vi "Change map display.vi"(9 "robot direction":string, 10 "robot location":dbl[](array[numeric]), 11 "Display Map":dbl[][](array[numeric])) -> (3 "New Display Map":dbl[][](array[numeric]))   [LabVIEW 2015]
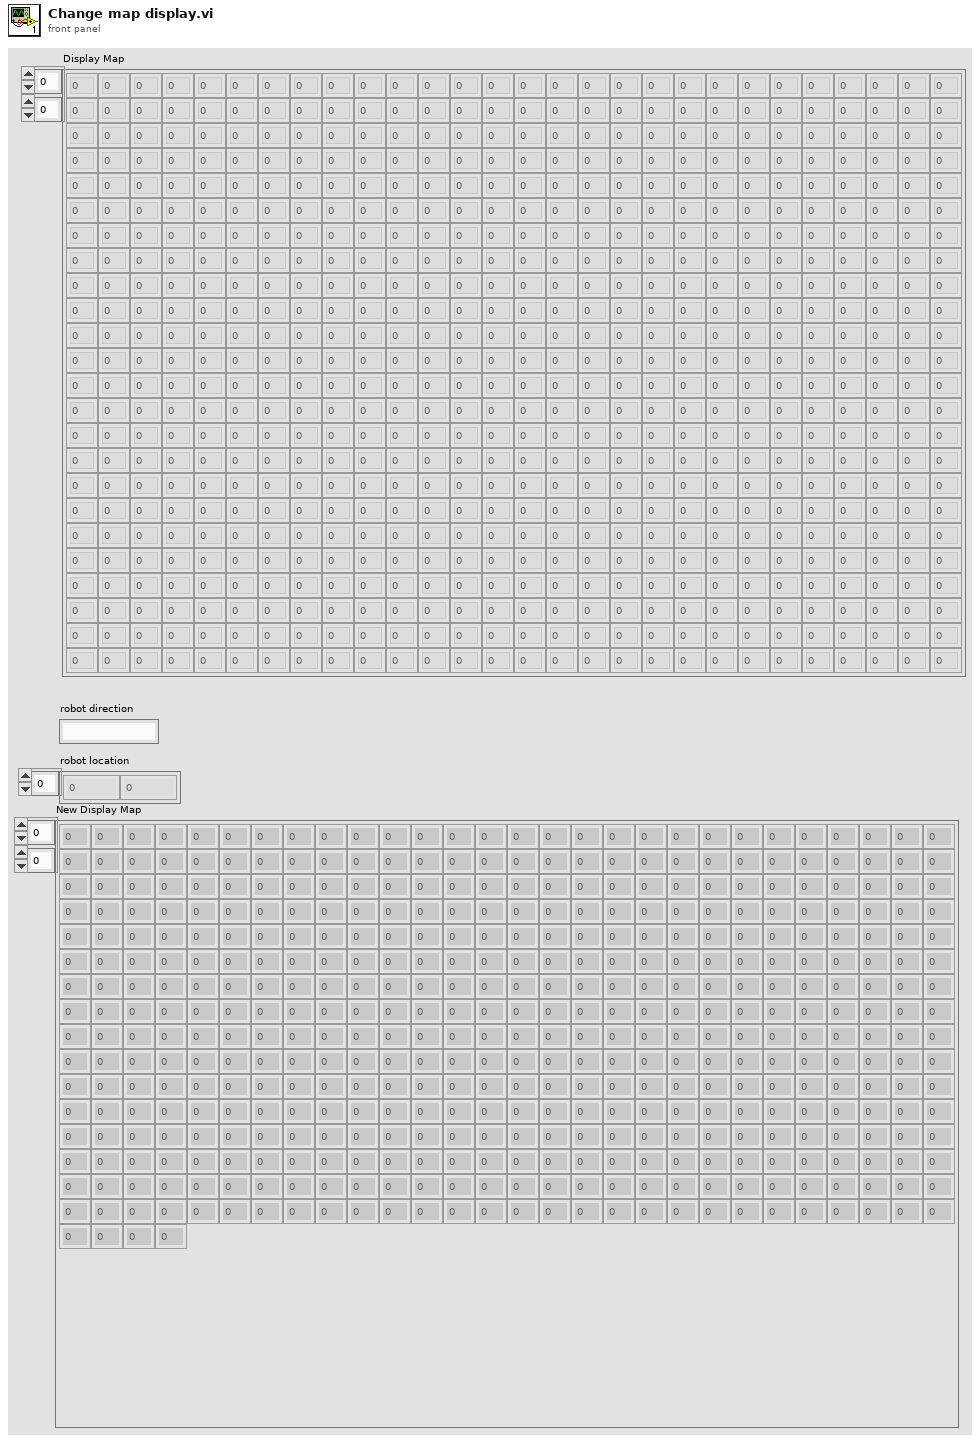
[diagram p1: front panel]
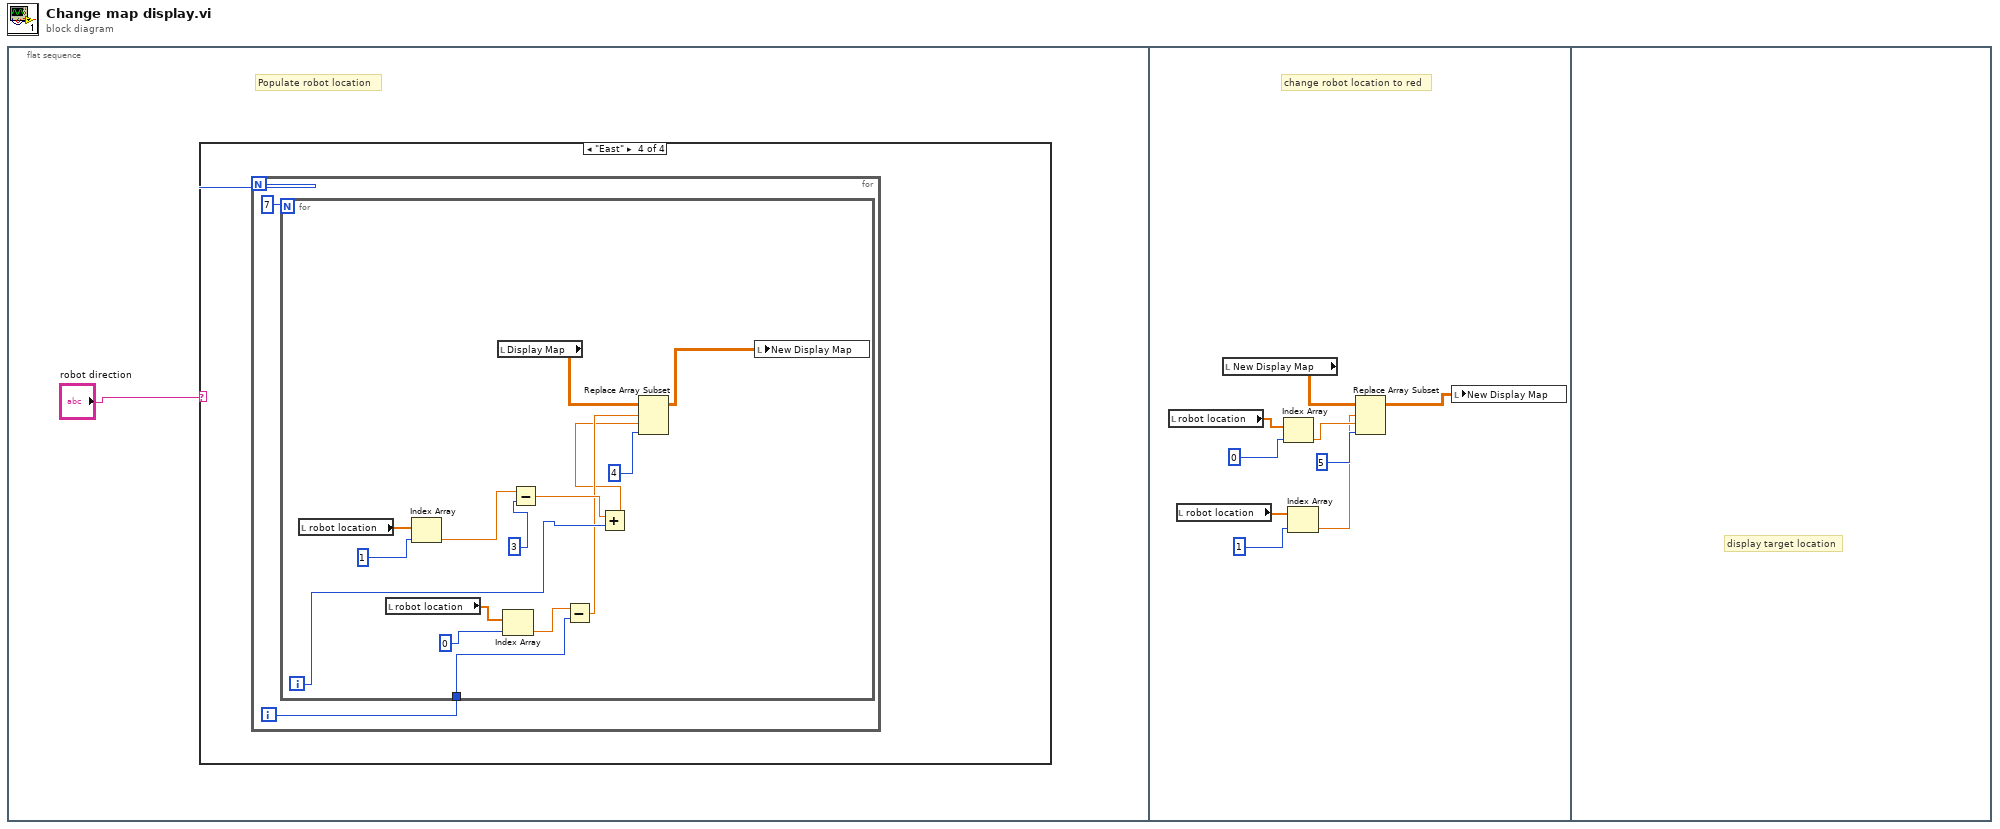
[diagram p0: block diagram]
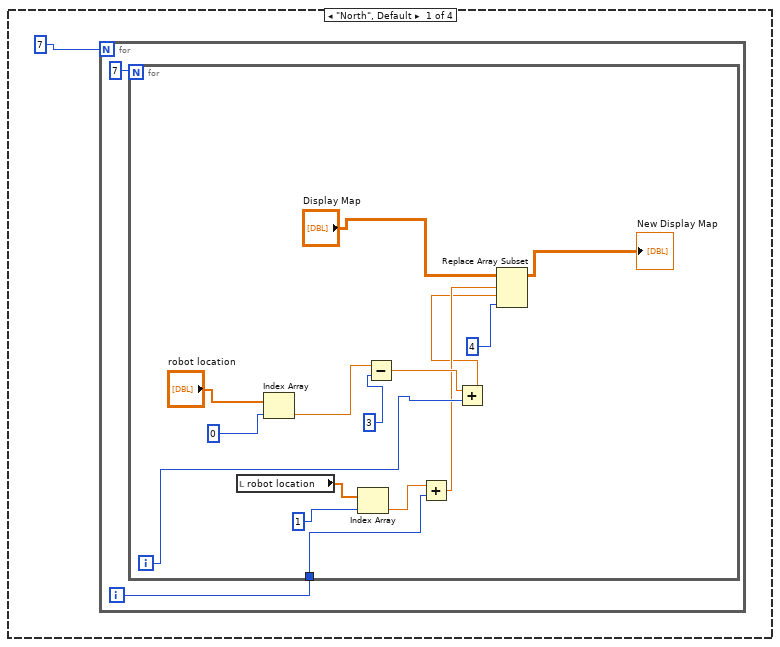
[diagram p2: hidden frame]
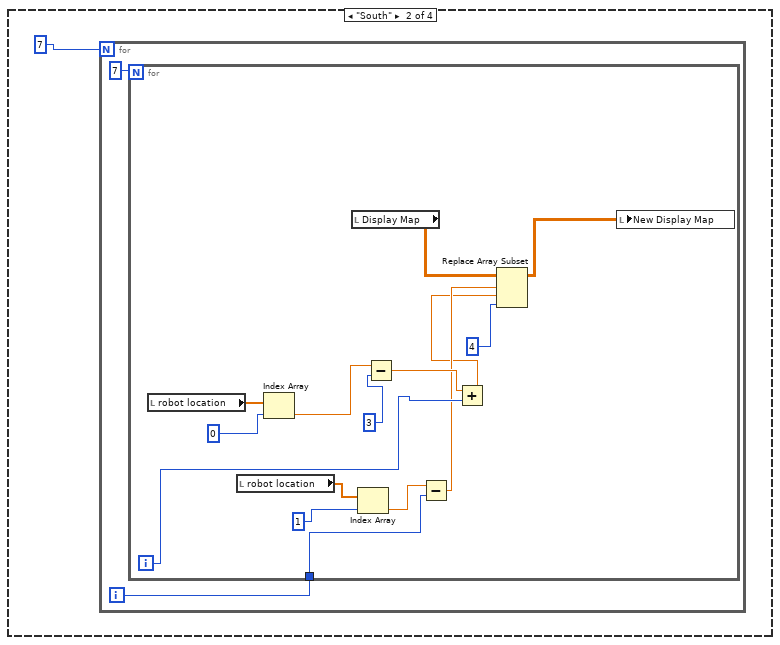
[diagram p3: hidden frame]
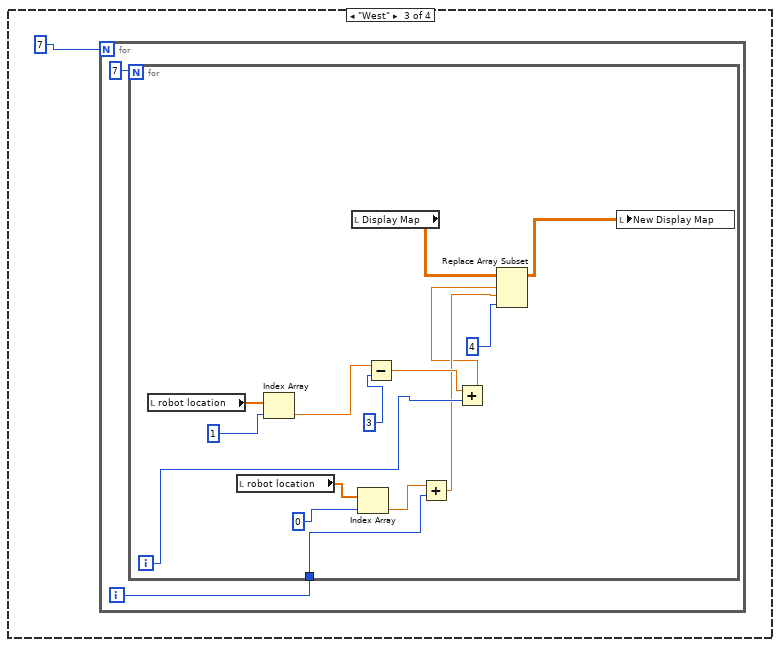
[diagram p4: hidden frame]
diagram:
  n1 = flat-sequence {
    frame #0 {
      # "Populate robot location"
      n2 = case shown="\"East\"" "robot direction" {
        frame "North", Default {
          n3 = for {
            N: 7 -> [_]
            i -> [w3]
            n4 = for {
              N: 7 -> [_]
              tunnel: w3 -> [w8]
              i -> [w12]
              n5 = local read "robot location"() -> (w17:dbl[])
              n6 = Index Array(array="robot location", index=0) -> (element=w14:dbl)
              n7 = Index Array(array=w17, index=1) -> (element=w15:dbl)
              n8 = Subtract(x=w14, y=3) -> (x-y=w11:dbl)
              n9 = Add(x=w15, y=w8) -> (x+y=w10:dbl)
              n10 = Add(x=w11, y=w12) -> (x+y=w9:dbl)
              n11 = Replace Array Subset(array="Display Map", new element=4, index (row)=w10, index (col)=w9) -> (→"New Display Map":dbl[][])
            }
          }
        }
        frame "South" {
          n12 = for {
            N: 7 -> [_]
            i -> [w21]
            n13 = for {
              N: 7 -> [_]
              tunnel: w21 -> [w23]
              i -> [w27]
              n14 = local read "robot location"() -> (w34:dbl[])
              n15 = local read "robot location"() -> (w32:dbl[])
              n16 = Index Array(array=w34, index=0) -> (element=w29:dbl)
              n17 = local read "Display Map"() -> (w37:dbl[][])
              n18 = Index Array(array=w32, index=1) -> (element=w30:dbl)
              n19 = Subtract(x=w29, y=3) -> (x-y=w26:dbl)
              n20 = Subtract(x=w30, y=w23) -> (x-y=w25:dbl)
              n21 = Add(x=w26, y=w27) -> (x+y=w24:dbl)
              n22 = Replace Array Subset(array=w37, new element=4, index (row)=w25, index (col)=w24) -> (w36:dbl[][])
              n23 = local write "New Display Map"(w36) -> ()
            }
          }
        }
        frame "West" {
          n24 = for {
            N: 7 -> [_]
            i -> [w39]
            n25 = for {
              N: 7 -> [_]
              tunnel: w39 -> [w43]
              i -> [w45]
              n26 = local read "robot location"() -> (w52:dbl[])
              n27 = local read "robot location"() -> (w50:dbl[])
              n28 = Index Array(array=w52, index=1) -> (element=w47:dbl)
              n29 = local read "Display Map"() -> (w55:dbl[][])
              n30 = Index Array(array=w50, index=0) -> (element=w48:dbl)
              n31 = Subtract(x=w47, y=3) -> (x-y=w44:dbl)
              n32 = Add(x=w48, y=w43) -> (x+y=w42:dbl)
              n33 = Add(x=w44, y=w45) -> (x+y=w41:dbl)
              n34 = Replace Array Subset(array=w55, new element=4, index (row)=w41, index (col)=w42) -> (w54:dbl[][])
              n35 = local write "New Display Map"(w54) -> ()
            }
          }
        }
        frame "East" {
          n36 = for {
            N: 7 -> [_]
            i -> [w57]
            n37 = for {
              N: 7 -> [_]
              tunnel: w57 -> [w62]
              i -> [w64]
              n38 = local read "robot location"() -> (w71:dbl[])
              n39 = local read "robot location"() -> (w69:dbl[])
              n40 = Index Array(array=w71, index=1) -> (element=w66:dbl)
              n41 = local read "Display Map"() -> (w61:dbl[][])
              n42 = Index Array(array=w69, index=0) -> (element=w67:dbl)
              n43 = Subtract(x=w66, y=3) -> (x-y=w63:dbl)
              n44 = Subtract(x=w67, y=w62) -> (x-y=w60:dbl)
              n45 = Add(x=w63, y=w64) -> (x+y=w59:dbl)
              n46 = Replace Array Subset(array=w61, new element=4, index (row)=w60, index (col)=w59) -> (w73:dbl[][])
              n47 = local write "New Display Map"(w73) -> ()
            }
          }
        }
      }
    }
    frame #1 {
      # "change robot location to red"
      n48 = local read "robot location"() -> (w80:dbl[])
      n49 = local read "robot location"() -> (w79:dbl[])
      n50 = local read "New Display Map"() -> (w78:dbl[][])
      n51 = Index Array(array=w80, index=0) -> (element=w81:dbl)
      n52 = Index Array(array=w79, index=1) -> (element=w76:dbl)
      n53 = Replace Array Subset(array=w78, new element=5, index (row)=w76, index (col)=w81) -> (w77:dbl[][])
      n54 = local write "New Display Map"(w77) -> ()
    }
    frame #2 {
      # "display target location"
    }
  }
